vi "route.vi"() -> ()   [LabVIEW 2014]
uses:
  <vilib>/Utility/sysdir.llb/System Directory Type.ctl
  <vilib>/Utility/config.llb/Read Key (Path).vi
  <vilib>/Utility/file.llb/Write To Spreadsheet File (string).vi
  <vilib>/Utility/config.llb/Write Key (Path).vi
  <vilib>/httpClient/LabVIEWHTTPClient.lvlib
  <vilib>/Utility/config.llb/NI_LVConfig.lvlib
panel:
  out "FUEL/연료":i32
  out "time/시간":dbl
  in  "도움말":bool
  in  "피드백":bool
  in  "저장 경로":path
  out "Distance":string="0"
  in  "찾기":bool
  in  "?":bool
  in  "?":bool
  out "x fmc 플랜":string
  out "FMS 플랜":string
  in  "Destination":string
  in  "departure":string
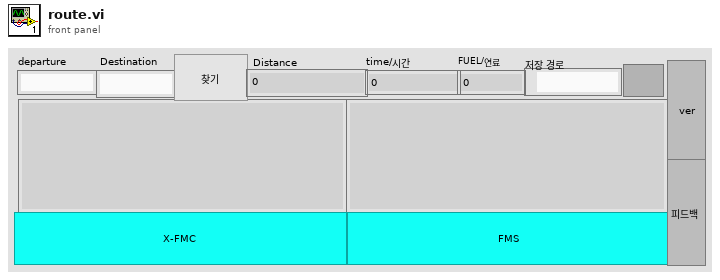
[diagram p1: front panel]
types:
  T1 = enum16{"open", "replace", "create", "open or create", "replace or create", "replace or create with confirmation"}
  T2 = typedef "System Directory Type.ctl" = i32
  T3 = typedef "NI_LVConfig.lvlib/Config Data RefNum.ctl" = refnum<k1>
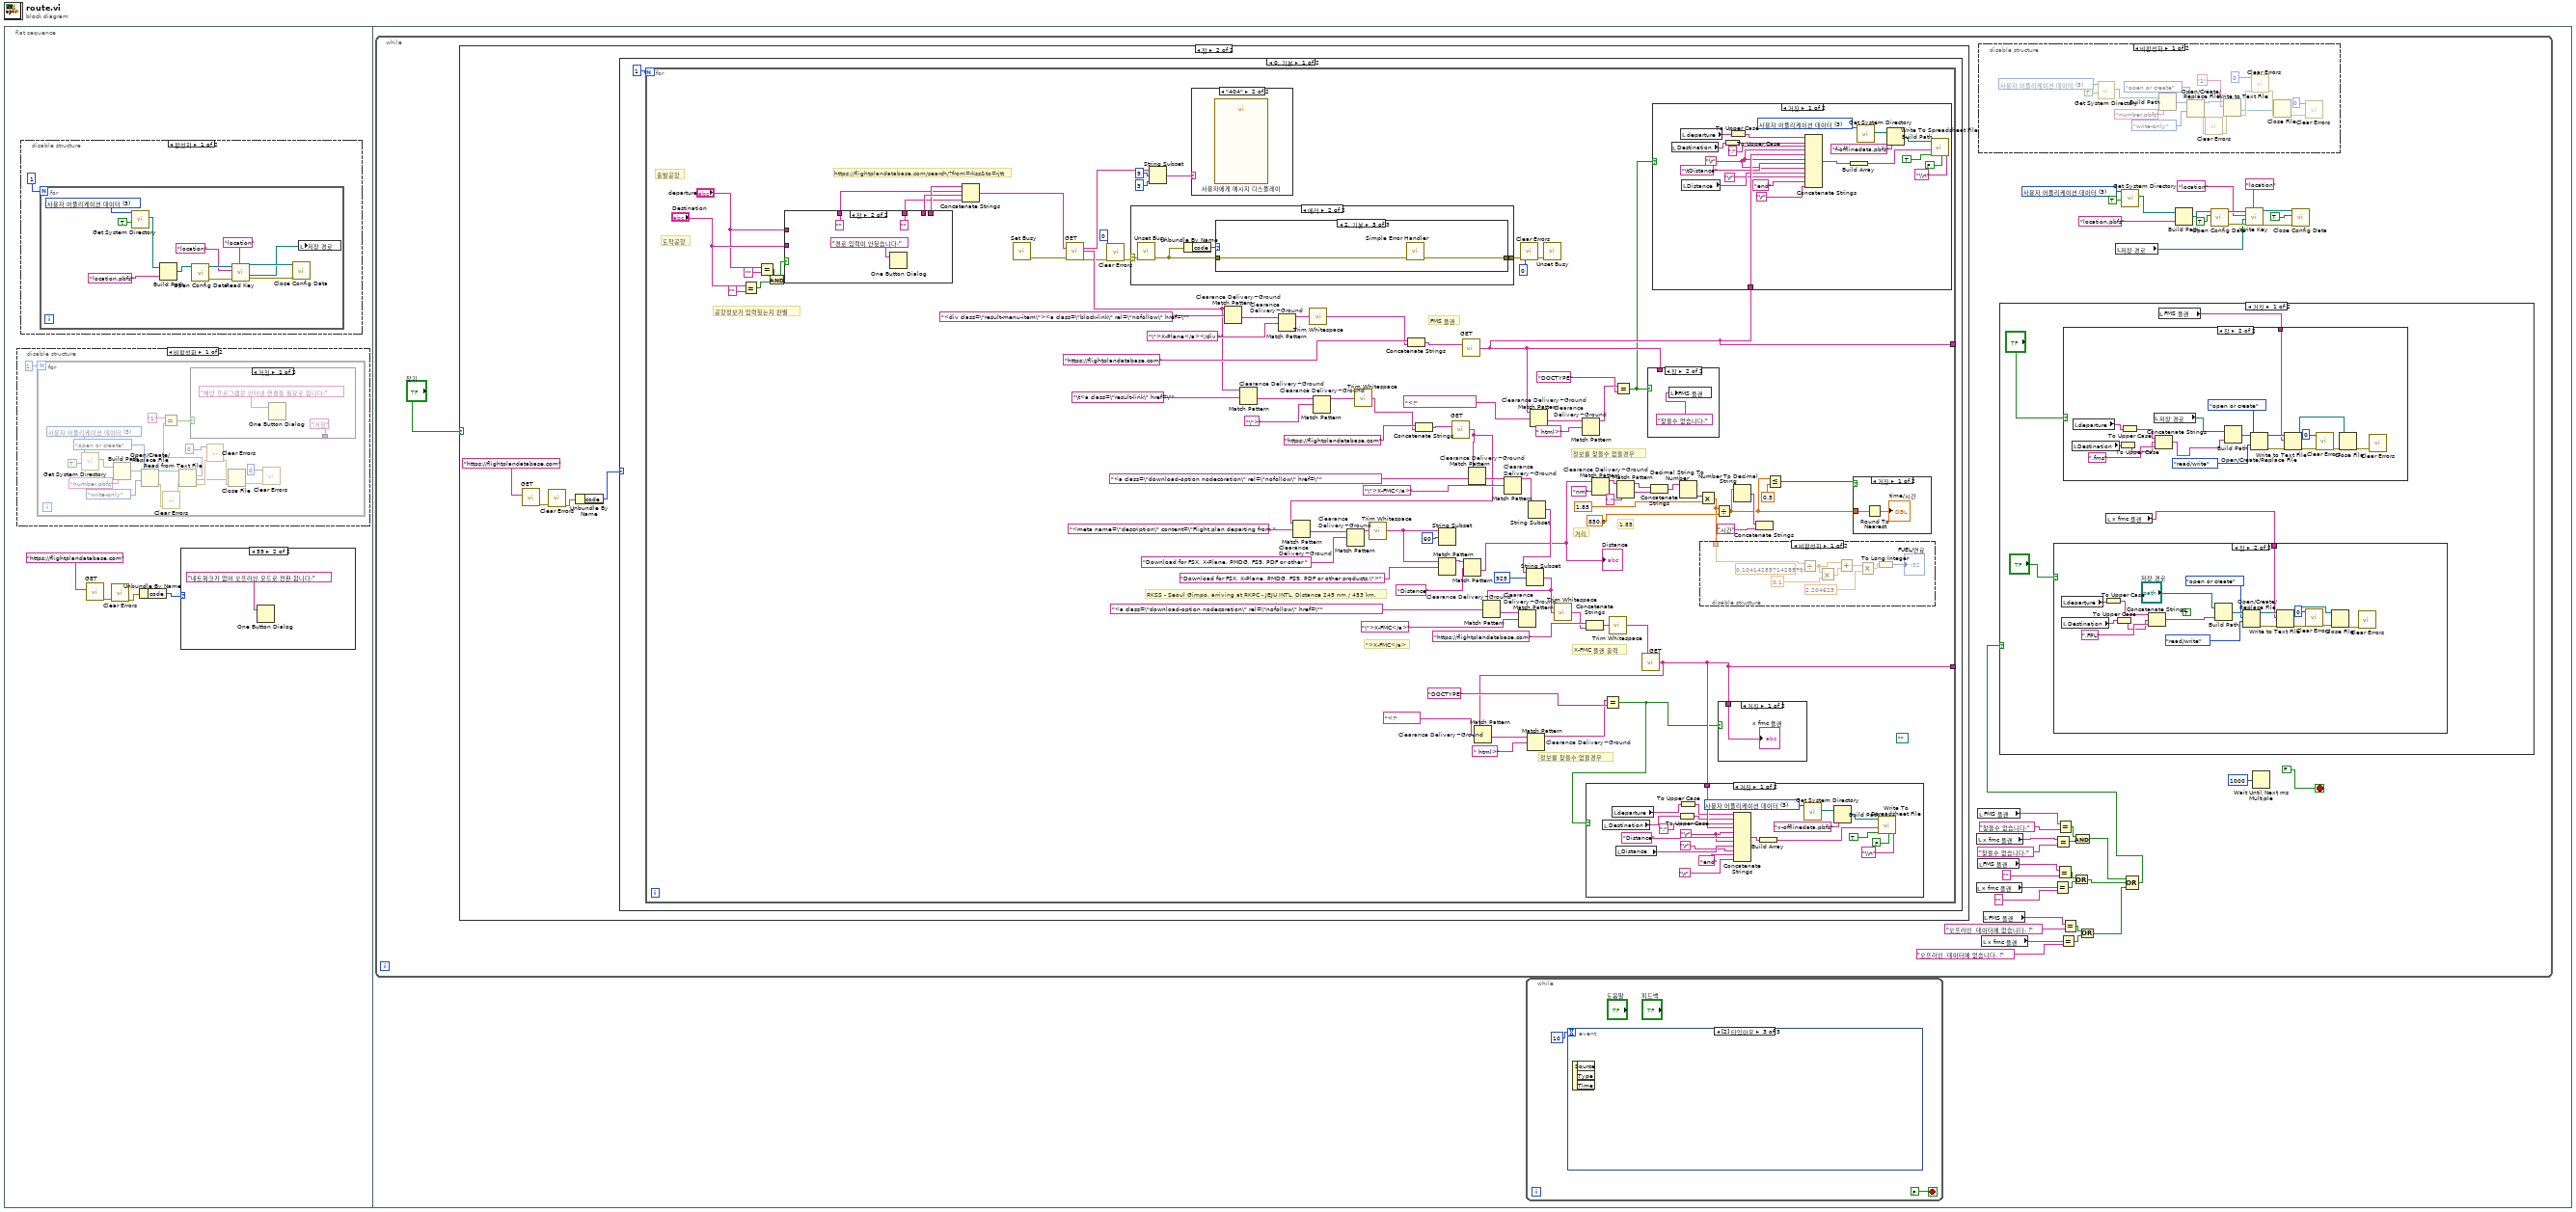
[diagram p0: block diagram]
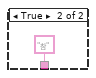
[diagram p3: hidden frame]
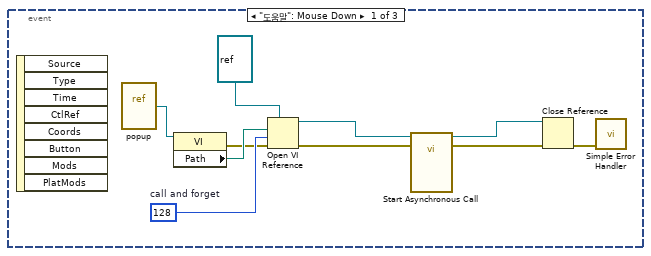
[diagram p6: hidden frame]
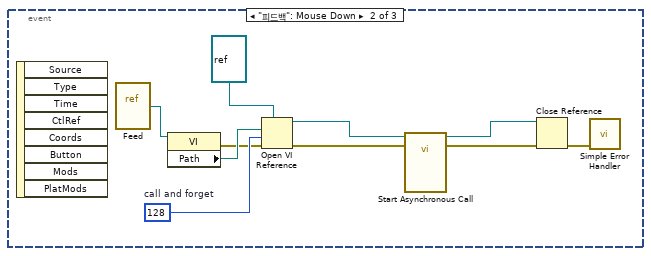
[diagram p7: hidden frame]
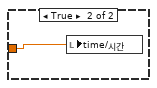
[diagram p12: hidden frame]
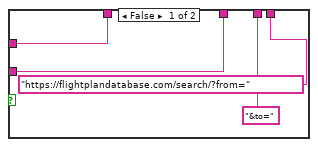
[diagram p13: hidden frame]
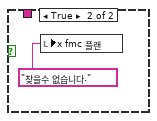
[diagram p14: hidden frame]
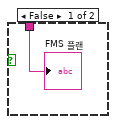
[diagram p15: hidden frame]
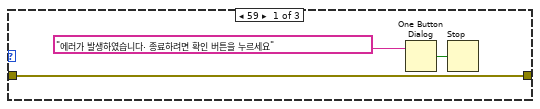
[diagram p18: hidden frame]
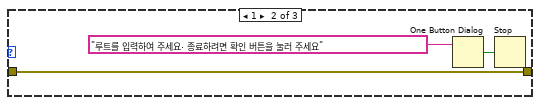
[diagram p19: hidden frame]
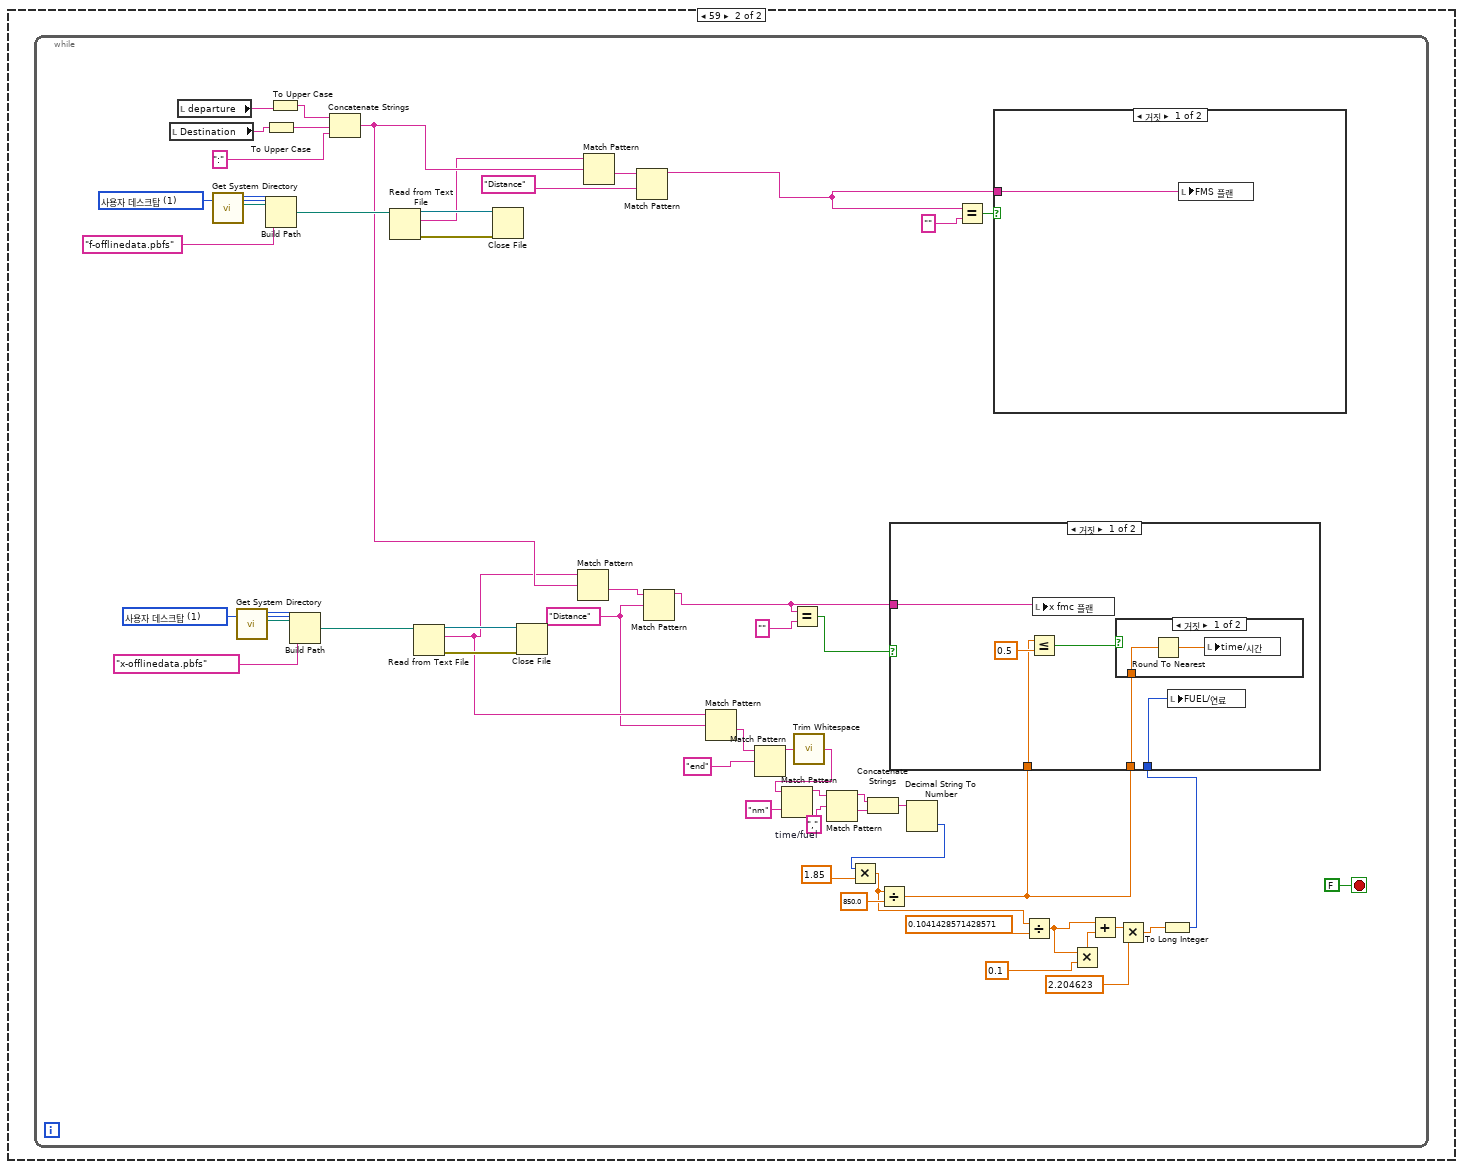
[diagram p20: hidden frame]
diagram:
  n1 = flat-sequence {
    frame #0 {
      n2 = disable-structure shown="비활성화" {
        frame Disabled {
          n3 = for {
            N: 1 -> [_]
            w12 = T2 3 items=["사용자 홈"=0, "사용자 데스크탑"=1, "사용자 문서"=2, "사용자 어플리케이션 데이터"=3, "사용자 환경"=4, "사용자 임시"=5, "퍼블릭 문서"=6, "퍼블릭 어플리케이션 데이터"=7, "퍼블릭 환경"=8, "퍼블릭 캐시"=13, "시스템 코어 라이브러리"=9, "시스템 설치된 라이브러리"=10, "어플리케이션 파일"=11, "부팅 볼륨 루트"=12] ("system directory type")
            n4 = call <vilib>:"Get System Directory.vi"("create directory if not found? (F)"=TRUE, "system directory type"=w12) -> ("system directory"=w13:path)  [unwired: 9 in]
            n5 = Build Path(base path=w13, name or relative path="number.pbfs" ("이름 또는 상대 경로")) -> (appended path=w18:path)
            n6 = Open/Create/Replace File(file path (use dialog)=w18, operation (0:open)=T1."open or create" ("동작(0:open)"), access (0:read/write)=enum16{"read/write", "read-only", "write-only"}."write-only" ("접근(0:읽기/쓰기)")) -> (refnum out=w21:refnum<file>, error out=w10:errorcluster)  [unwired: 3 in, 1 out]
            n7 = call <vilib>:"Clear Errors.vi"("error in (no error)"=w10) -> ("error out"=w9:errorcluster)  [unwired: 5 in, 1 out]
            n8 = Read from Text File(file (use dialog)=w21, error in=w9) -> (refnum out=w22:refnum<file>, text=w7:string, error out=w23:errorcluster)  [unwired: 2 in, 1 out]
            n9 = Equal?(x="1" ("y"), y=w7) -> (x = y?=w17:bool)
            n10 = case shown="거짓" w17 {
              tunnel: ["거짓" "참"] -> _
              frame False {
                n11 = One Button Dialog(message="해당 프로그램은 인터넷 연결을 필요로 합니다." ("메시지")) -> ()  [unwired: 1 in, 1 out]
              }
              frame True {
              }
            }
            n12 = call <vilib>:"Clear Errors.vi"("error in (no error)"=w23, "specific error code to clear (0: all)"=0) -> ("error out"=w24:errorcluster)  [unwired: 4 in, 1 out]
            n13 = Close File(refnum=w22, error in=w24) -> (error out=w15:errorcluster)  [unwired: 1 out]
            n14 = call <vilib>:"Clear Errors.vi"("error in (no error)"=w15, "specific error code to clear (0: all)"=0) -> ()  [unwired: 4 in, 2 out]
          }
        }
        frame Enabled {
        }
      }
      n15 = disable-structure shown="활성화" {
        frame Enabled {
          n16 = for {
            N: 1 -> [_]
            w40 = T2 3 items=["사용자 홈"=0, "사용자 데스크탑"=1, "사용자 문서"=2, "사용자 어플리케이션 데이터"=3, "사용자 환경"=4, "사용자 임시"=5, "퍼블릭 문서"=6, "퍼블릭 어플리케이션 데이터"=7, "퍼블릭 환경"=8, "퍼블릭 캐시"=13, "시스템 코어 라이브러리"=9, "시스템 설치된 라이브러리"=10, "어플리케이션 파일"=11, "부팅 볼륨 루트"=12] ("system directory type")
            n17 = call <vilib>:"Get System Directory.vi"("create directory if not found? (F)"=TRUE, "system directory type"=w40) -> ("system directory"=w38:path)  [unwired: 9 in]
            n18 = Build Path(base path=w38, name or relative path="location.pbfs" ("문자열")) -> (appended path=w37:path)
            n19 = call <vilib>:"Open Config Data.vi"("configuration file path"=w37) -> ("error out"=w34:errorcluster, "refnum"=w33:T3)  [unwired: 8 in, 1 out]
            n20 = call-poly <vilib>:"Read Key.vi"("section"="location", "error in (no error)"=w34, "key"="location", "refnum"=w33) -> ("error out"=w35:errorcluster, "value"=w30:path, "refnum out"=w36:T3)  [unwired: 4 in, 1 out]
            n21 = call <vilib>:"Close Config Data.vi"("error in (no error)"=w35, "refnum"=w36) -> ()  [unwired: 8 in, 2 out]
            n22 = local write "저장 경로"(w30) -> ()
          }
        }
        frame Disabled {
        }
      }
      n23 = call <vilib>:"GET.vi"("url"="https://flightplandatabase.com") -> ("error out"=w4:errorcluster)  [unwired: 11 in, 3 out]
      n24 = call <vilib>:"Clear Errors.vi"("error in (no error)"=w4) -> ("error out"=w2:errorcluster)  [unwired: 5 in, 1 out]
      n25 = Unbundle By Name(w2) -> ("code"=w1:i32)
      n26 = case shown="59" w1 {
        frame 0, Default {
        }
        frame 59 {
          n27 = One Button Dialog(message="네트워크가 없어 오프라인 모드로 전환 합니다." ("메시지")) -> ()  [unwired: 1 in, 1 out]
        }
      }
    }
    frame #1 {
      n28 = while {
        stop <- FALSE stop-if-true
        w84 = T2 3 items=["사용자 홈"=0, "사용자 데스크탑"=1, "사용자 문서"=2, "사용자 어플리케이션 데이터"=3, "사용자 환경"=4, "사용자 임시"=5, "퍼블릭 문서"=6, "퍼블릭 어플리케이션 데이터"=7, "퍼블릭 환경"=8, "퍼블릭 캐시"=13, "시스템 코어 라이브러리"=9, "시스템 설치된 라이브러리"=10, "어플리케이션 파일"=11, "부팅 볼륨 루트"=12] ("system directory type")
        n29 = case shown="참" "찾기" {
          frame False {
          }
          frame True {
            n30 = call <vilib>:"GET.vi"("url"="https://flightplandatabase.com") -> ("error out"=w106:errorcluster)  [unwired: 11 in, 3 out]
            n31 = call <vilib>:"Clear Errors.vi"("error in (no error)"=w106) -> ("error out"=w104:errorcluster)  [unwired: 5 in, 1 out]
            n32 = Unbundle By Name(w104) -> ("code"=w103:i32)
            n33 = case shown="0, 기본" w103 {
              frame 0, Default {
                n34 = for {
                  N: 1 -> [_]
                  tunnel: [w111] -> _
                  tunnel: [w109] -> _
                  (unwired) path ""
                  # "1.85"
                  # "RKSS - Seoul Gimpo, arriving at RKPC - JEJU INTL. Distance 245 nm / 453 km."
                  # "\">X-FMC</a>"
                  # "https://flightplandatabase.com/search/?from=rkss&to=rjtt"
                  # "FMS 플랜"
                  # "거리"
                  # "X-FMC 플랜 출력"
                  # "정보를 찾을수 없을경우"
                  # "정보를 찾을수 없을경우"
                  # "공항정보가 입력됫는지 판별"
                  # "도착공항"
                  # "출발공항"
                  n35 = Equal?(x="Destination", y="") -> (x = y?=w139:bool)
                  n36 = Equal?(x="departure", y="") -> (x = y?=w138:bool)
                  n37 = And(x=w138, y=w139) -> (x .and. y?=w140:bool)
                  n38 = case shown="참" w140 {
                    tunnel: ["&to=" ("문자열") _] -> w129
                    tunnel: ["https://flightplandatabase.com/search/?from=" ("문자열") _] -> w128
                    tunnel: "Destination" -> [w255 _]
                    tunnel: [w255 "" ("Destination")] -> w126
                    tunnel: [w254 "" ("departure")] -> w124
                    tunnel: "departure" -> [w254 _]
                    frame False {
                    }
                    frame True {
                      n39 = One Button Dialog(message="경로 입력이 안됫습니다." ("메시지")) -> ()  [unwired: 1 in, 1 out]
                    }
                  }
                  n40 = Concatenate Strings(w128, w124, w129, w126) -> (w190:string)
                  n41 = call <vilib>:"Set Busy.vi"() -> ("error out"=w195:errorcluster)  [unwired: 10 in, 1 out]
                  n42 = call <vilib>:"GET.vi"("url"=w190, "error in (no error)"=w195) -> ("headers"=w199:string, "body"=w166:string, "error out"=w149:errorcluster)  [unwired: 10 in, 1 out]
                  n43 = call <vilib>:"Clear Errors.vi"("error in (no error)"=w149, "specific error code to clear (0: all)"=0) -> ("error out"=w150:errorcluster)  [unwired: 4 in, 1 out]
                  n44 = case shown="에러" w150 {
                    selector: w150 -> [w265 w268]
                    tunnel: [w265 w266] -> w146
                    frame No Error {
                    }
                    frame Error {
                      n45 = call <vilib>:"Unset Busy.vi"("error in (no error)"=w268) -> ("error out"=w267:errorcluster)  [unwired: 10 in]
                      n46 = Unbundle By Name(w267) -> ("code"=w269:i32)
                      n47 = case shown="2, 기본" w269 {
                        tunnel: w267 -> [w270 w275 w277]
                        tunnel: [w270 w275 w276] -> w266
                        frame 59 {
                          n48 = One Button Dialog(message="에러가 발생하였습니다. 종료하려면 확인 버튼을 누르세요" ("메시지")) -> (true=w271:bool)  [unwired: 1 in]
                          n49 = Stop(stop? (T)=w271) -> ()
                        }
                        frame 1 {
                          n50 = One Button Dialog(message="루트를 입력하여 주세요. 종료하려면 확인 버튼을 눌러 주세요" ("메시지")) -> (true=w273:bool)  [unwired: 1 in]
                          n51 = Stop(stop? (T)=w273) -> ()
                        }
                        frame 2, Default {
                          n52 = call <vilib>:"Simple Error Handler.vi"("error in (no error)"=w277) -> ("error out"=w276:errorcluster)  [unwired: 4 in, 4 out]
                        }
                      }
                    }
                  }
                  n53 = String Subset(string=w199, offset (0)=9 ("오프셋(0)"), length (rest)=3 ("길이(나머지)")) -> (substring=w196:string)
                  n54 = case shown="\"404\"" w196 {
                    frame "거짓", Default {
                    }
                    frame "404" {
                      n55 = call "사용자에게 메시지 디스플레이"() -> ()  [unwired: 10 in, 2 out]
                    }
                  }
                  n56 = Match Pattern "Clearance Delivery~Ground"(string=w166, regular expression="<div class=\"result-menu-item\"><a class=\"block-link\" rel=\"nofollow\" href=\"" ("정규식")) -> (after substring=w193:string)  [unwired: 1 in, 3 out]
                  n57 = Match Pattern "Clearance Delivery~Ground"(string=w166, regular expression="\t<a class=\"result-link\" href=\"" ("정규식")) -> (after substring=w186:string)  [unwired: 1 in, 3 out]
                  n58 = Match Pattern "Clearance Delivery~Ground"(string=w193, regular expression="\">X-Plane</a></div>" ("정규식")) -> (before substring=w191:string)  [unwired: 1 in, 3 out]
                  n59 = call <vilib>:"Trim Whitespace.vi"("string"=w191) -> ("trimmed string"=w187:string)  [unwired: 1 in]
                  n60 = Match Pattern "Clearance Delivery~Ground"(string=w186, regular expression="\">" ("정규식")) -> (before substring=w183:string)  [unwired: 1 in, 3 out]
                  n61 = call <vilib>:"Trim Whitespace.vi"("string"=w183) -> ("trimmed string"=w181:string)  [unwired: 1 in]
                  n62 = Concatenate Strings("https://flightplandatabase.com" ("url"), w187) -> (w188:string)
                  n63 = Concatenate Strings("https://flightplandatabase.com" ("url"), w181) -> (w178:string)
                  n64 = call <vilib>:"GET.vi"("url"=w178) -> ("body"=w164:string)  [unwired: 11 in, 3 out]
                  n65 = Match Pattern "Clearance Delivery~Ground"(string=w164, regular expression="<meta name=\"description\" content=\"Flight plan departing from " ("정규식")) -> (after substring=w167:string)  [unwired: 1 in, 3 out]
                  n66 = Match Pattern "Clearance Delivery~Ground"(string=w167, regular expression="Download for FSX, X-Plane, PMDG, FS9, PDF or other " ("정규식")) -> (before substring=w169:string)  [unwired: 1 in, 3 out]
                  n67 = call <vilib>:"Trim Whitespace.vi"("string"=w169) -> ("trimmed string"=w134:string)  [unwired: 1 in]
                  n68 = String Subset(string=w134, offset (0)=60 ("오프셋(0)")) -> ()  [unwired: 1 in, 1 out]
                  n69 = Match Pattern(string=w134, regular expression="Download for FSX, X-Plane, PMDG, FS9, PDF or other products.\">" ("정규식")) -> (before substring=w132:string)  [unwired: 1 in, 3 out]
                  n70 = call <vilib>:"GET.vi"("url"=w188) -> ("body"=w109:string)  [unwired: 11 in, 3 out]
                  n71 = Match Pattern(string=w132, regular expression="Distance" ("정규식")) -> (after substring=w130:string)  [unwired: 1 in, 3 out]
                  "Distance" <- w130
                  n72 = Match Pattern "Clearance Delivery~Ground"(string=w164, regular expression="<a class=\"download-option nodecoration\" rel=\"nofollow\" href=\"" ("정규식")) -> (after substring=w177:string)  [unwired: 1 in, 3 out]
                  n73 = Match Pattern "Clearance Delivery~Ground"(string=w177, regular expression="\">X-FMC</a>" ("정규식")) -> (before substring=w176:string)  [unwired: 1 in, 3 out]
                  n74 = call <vilib>:"Clear Errors.vi"("error in (no error)"=w146, "specific error code to clear (0: all)"=0) -> ("error out"=w147:errorcluster)  [unwired: 4 in, 1 out]
                  n75 = String Subset(string=w176) -> (substring=w135:string)  [unwired: 2 in]
                  n76 = String Subset(string=w135, offset (0)=925 ("오프셋(0)")) -> (substring=w136:string)  [unwired: 1 in]
                  n77 = Match Pattern "Clearance Delivery~Ground"(string=w136, regular expression="<a class=\"download-option nodecoration\" rel=\"nofollow\" href=\"" ("정규식")) -> (after substring=w173:string)  [unwired: 1 in, 3 out]
                  n78 = Match Pattern "Clearance Delivery~Ground"(string=w173, regular expression="\">X-FMC</a>" ("정규식")) -> ()  [unwired: 1 in, 4 out]
                  n79 = Match Pattern "Clearance Delivery~Ground"(string=w109, regular expression="<!" ("문자열")) -> (after substring=w161:string)  [unwired: 1 in, 3 out]
                  n80 = call <vilib>:"Unset Busy.vi"("error in (no error)"=w147) -> ()  [unwired: 10 in, 1 out]
                  n81 = call <vilib>:"Trim Whitespace.vi"("string"=w136) -> ("trimmed string"=w171:string)  [unwired: 1 in]
                  n82 = Match Pattern "Clearance Delivery~Ground"(string=w161, regular expression=" html>" ("정규식")) -> (before substring=w160:string)  [unwired: 1 in, 3 out]
                  n83 = Concatenate Strings("https://flightplandatabase.com" ("url"), w171) -> (w170:string)
                  n84 = Match Pattern "Clearance Delivery~Ground"(string=w130, regular expression="nm" ("정규식")) -> (before substring=w120:string)  [unwired: 1 in, 3 out]
                  n85 = call <vilib>:"Trim Whitespace.vi"("string"=w170) -> ("trimmed string"=w153:string)  [unwired: 1 in]
                  n86 = Equal?(x=w160, y="DOCTYPE") -> (x = y?=w108:bool)
                  n87 = Match Pattern(string=w120, regular expression="," ("정규식")) -> (before substring=w117:string, after substring=w116:string)  [unwired: 1 in, 2 out]
                  n88 = call <vilib>:"GET.vi"("url"=w153) -> ("body"=w111:string)  [unwired: 11 in, 3 out]
                  n89 = Match Pattern "Clearance Delivery~Ground"(string=w111, regular expression="<!" ("문자열")) -> (after substring=w158:string)  [unwired: 1 in, 3 out]
                  n90 = Match Pattern "Clearance Delivery~Ground"(string=w158, regular expression=" html>" ("정규식")) -> (before substring=w155:string)  [unwired: 1 in, 3 out]
                  n91 = Equal?(x=w155, y="DOCTYPE") -> (x = y?=w110:bool)
                  n92 = case shown="거짓" w110 {
                    tunnel: w111 -> [w240 _]
                    frame False {
                      w234 = "\r"
                      w243 = T2 3 items=["사용자 홈"=0, "사용자 데스크탑"=1, "사용자 문서"=2, "사용자 어플리케이션 데이터"=3, "사용자 환경"=4, "사용자 임시"=5, "퍼블릭 문서"=6, "퍼블릭 어플리케이션 데이터"=7, "퍼블릭 환경"=8, "퍼블릭 캐시"=13, "시스템 코어 라이브러리"=9, "시스템 설치된 라이브러리"=10, "어플리케이션 파일"=11, "부팅 볼륨 루트"=12] ("system directory type")
                      n93 = local read "Destination"() -> (w236:string)
                      n94 = local read "departure"() -> (w239:string)
                      n95 = local read "Distance"() -> (w233:string)
                      n96 = To Upper Case(1:w236) -> (0:w237:string)
                      n97 = To Upper Case(1:w239) -> (0:w238:string)
                      n98 = Concatenate Strings(w238, w237, ":", w240, w234, "Distance" ("문자열"), w234, w233, "\r", "end", "\r") -> (w241:string)
                      n99 = Build Array(w241) -> (w245:string[])
                      n100 = call <vilib>:"Get System Directory.vi"("system directory type"=w243) -> ("system directory"=w247:path)  [unwired: 10 in]
                      n101 = Build Path(base path=w247, name or relative path="x-offlinedata.pbfs" ("이름 또는 상대 경로")) -> (appended path=w246:path)
                      n102 = call-poly <vilib>:"Write To Spreadsheet File.vi"("delimiter (\\t)"="\\n" ("delimiter (\\t)"), "transpose? (no:F)"=FALSE, "append to file? (new file:F)"=TRUE, "1D data"=w245, "file path (dialog if empty)"=w246) -> ()  [unwired: 3 in, 1 out]
                    }
                    frame True {
                    }
                  }
                  n103 = case shown="참" w108 {
                    tunnel: w109 -> [w263 _]
                    frame False {
                      "FMS 플랜" <- w263
                    }
                    frame True {
                      n104 = local write "FMS 플랜"("찾을수 없습니다.") -> ()
                    }
                  }
                  n105 = Concatenate Strings(w117, w116) -> (w119:string)
                  n106 = case shown="거짓" w108 {
                    tunnel: w109 -> [w215 _]
                    frame False {
                      w213 = "\r"
                      w222 = T2 3 items=["사용자 홈"=0, "사용자 데스크탑"=1, "사용자 문서"=2, "사용자 어플리케이션 데이터"=3, "사용자 환경"=4, "사용자 임시"=5, "퍼블릭 문서"=6, "퍼블릭 어플리케이션 데이터"=7, "퍼블릭 환경"=8, "퍼블릭 캐시"=13, "시스템 코어 라이브러리"=9, "시스템 설치된 라이브러리"=10, "어플리케이션 파일"=11, "부팅 볼륨 루트"=12] ("system directory type")
                      n107 = local read "Destination"() -> (w216:string)
                      n108 = local read "departure"() -> (w218:string)
                      n109 = local read "Distance"() -> (w212:string)
                      n110 = To Upper Case(1:w216) -> (0:w217:string)
                      n111 = To Upper Case(1:w218) -> (0:w219:string)
                      n112 = Concatenate Strings(w219, w217, ":", w213, w215, w213, "\tDistance", w213, w212, "\r", "end", "\r") -> (w220:string)
                      n113 = Build Array(w220) -> (w224:string[])
                      n114 = call <vilib>:"Get System Directory.vi"("system directory type"=w222) -> ("system directory"=w226:path)  [unwired: 10 in]
                      n115 = Build Path(base path=w226, name or relative path="f-offlinedata.pbfs" ("이름 또는 상대 경로")) -> (appended path=w225:path)
                      n116 = call-poly <vilib>:"Write To Spreadsheet File.vi"("delimiter (\\t)"="\\n" ("delimiter (\\t)"), "transpose? (no:F)"=FALSE, "append to file? (new file:F)"=TRUE, "1D data"=w224, "file path (dialog if empty)"=w225) -> ()  [unwired: 3 in, 1 out]
                    }
                    frame True {
                    }
                  }
                  n117 = Decimal String To Number(string=w119) -> (number=w121:i32)  [unwired: 2 in, 1 out]
                  n118 = Multiply(x=w121, y=1.85) -> (x*y=w112:dbl)
                  n119 = disable-structure shown="비활성화" {
                    disable-tunnel: w112 -> [w205 _]
                    frame Disabled {
                      n120 = Divide(x=w205, y=0.1041428571428571) -> (x/y=w206:dbl)
                      n121 = Multiply(x=w206, y=0.1) -> (x*y=w204:dbl)
                      n122 = Add(x=w206, y=w204) -> (x+y=w203:dbl)
                      n123 = Multiply(x=w203, y=2.204623) -> (x*y=w200:dbl)
                      n124 = To Long Integer(number=w200) -> (32bit integer=→"FUEL/연료":i32)
                    }
                    frame Enabled {
                    }
                  }
                  n125 = Divide(x=w112, y=850.0) -> (x/y=w113:dbl)
                  n126 = case shown="거짓" w110 {
                    tunnel: w111 -> [w261 _]
                    frame False {
                      "x fmc 플랜" <- w261
                    }
                    frame True {
                      n127 = local write "x fmc 플랜"("찾을수 없습니다.") -> ()
                    }
                  }
                  n128 = Number To Decimal String(number=w113) -> (decimal integer string=w141:string)  [unwired: 1 in]
                  n129 = Concatenate Strings(w141, "시간") -> ()  [unwired: 1 out]
                  n130 = Less Or Equal?(x=w113, y=0.5) -> (x <= y?=w115:bool)
                  n131 = case shown="거짓" w115 {
                    tunnel: w113 -> [w252 w253]
                    frame False {
                      n132 = Round To Nearest(number=w252) -> (nearest integer value=→"time/시간":dbl)
                    }
                    frame True {
                      n133 = local write "time/시간"(w253) -> ()
                    }
                  }
                }
              }
              frame 59 {
                n134 = while {
                  stop <- FALSE stop-if-true
                  w278 = "Distance" ("정규식")
                  w315 = T2 1 items=["사용자 홈"=0, "사용자 데스크탑"=1, "사용자 문서"=2, "사용자 어플리케이션 데이터"=3, "사용자 환경"=4, "사용자 임시"=5, "퍼블릭 문서"=6, "퍼블릭 어플리케이션 데이터"=7, "퍼블릭 환경"=8, "퍼블릭 캐시"=13, "시스템 코어 라이브러리"=9, "시스템 설치된 라이브러리"=10, "어플리케이션 파일"=11, "부팅 볼륨 루트"=12] ("system directory type")
                  w329 = T2 1 items=["사용자 홈"=0, "사용자 데스크탑"=1, "사용자 문서"=2, "사용자 어플리케이션 데이터"=3, "사용자 환경"=4, "사용자 임시"=5, "퍼블릭 문서"=6, "퍼블릭 어플리케이션 데이터"=7, "퍼블릭 환경"=8, "퍼블릭 캐시"=13, "시스템 코어 라이브러리"=9, "시스템 설치된 라이브러리"=10, "어플리케이션 파일"=11, "부팅 볼륨 루트"=12] ("system directory type")
                  n135 = local read "Destination"() -> (w309:string)
                  n136 = local read "departure"() -> (w311:string)
                  n137 = call <vilib>:"Get System Directory.vi"("system directory type"=w315) -> ("system directory"=w314:path)  [unwired: 10 in]
                  n138 = call <vilib>:"Get System Directory.vi"("system directory type"=w329) -> ("system directory"=w330:path)  [unwired: 10 in]
                  n139 = To Upper Case(1:w309) -> (0:w308:string)
                  n140 = Build Path(base path=w314, name or relative path="f-offlinedata.pbfs" ("이름 또는 상대 경로")) -> (appended path=w317:path)
                  n141 = To Upper Case(1:w311) -> (0:w310:string)
                  n142 = Build Path(base path=w330, name or relative path="x-offlinedata.pbfs" ("이름 또는 상대 경로")) -> (appended path=w327:path)
                  n143 = Concatenate Strings(w310, w308, ":") -> (w305:string)
                  n144 = Read from Text File(file (use dialog)=w317) -> (refnum out=w318:refnum<file>, text=w303:string, error out=w319:errorcluster)  [unwired: 3 in, 1 out]
                  n145 = Read from Text File(file (use dialog)=w327) -> (refnum out=w326:refnum<file>, text=w279:string, error out=w325:errorcluster)  [unwired: 3 in, 1 out]
                  n146 = Close File(refnum=w318, error in=w319) -> ()  [unwired: 2 out]
                  n147 = Close File(refnum=w326, error in=w325) -> ()  [unwired: 2 out]
                  n148 = Match Pattern(string=w279, regular expression=w305) -> (after substring=w307:string)  [unwired: 1 in, 3 out]
                  n149 = Match Pattern(string=w303, regular expression=w305) -> (after substring=w312:string)  [unwired: 1 in, 3 out]
                  n150 = Match Pattern(string=w312, regular expression="Distance") -> (before substring=w313:string)  [unwired: 1 in, 3 out]
                  n151 = Match Pattern(string=w307, regular expression=w278) -> (before substring=w306:string)  [unwired: 1 in, 3 out]
                  n152 = Match Pattern(string=w279, regular expression=w278) -> (after substring=w302:string)  [unwired: 1 in, 3 out]
                  n153 = Match Pattern(string=w302, regular expression="end" ("정규식")) -> (before substring=w292:string)  [unwired: 1 in, 3 out]
                  n154 = Equal?(x=w306, y="") -> (x = y?=w324:bool)
                  n155 = call <vilib>:"Trim Whitespace.vi"("string"=w292) -> ("trimmed string"=w298:string)  [unwired: 1 in]
                  n156 = Match Pattern "time/fuel"(string=w298, regular expression="nm" ("정규식")) -> (before substring=w294:string)  [unwired: 1 in, 3 out]
                  n157 = Match Pattern(string=w294, regular expression="," ("정규식")) -> (before substring=w296:string, after substring=w297:string)  [unwired: 1 in, 2 out]
                  n158 = Concatenate Strings(w296, w297) -> (w295:string)
                  n159 = Decimal String To Number(string=w295) -> (number=w283:i32)  [unwired: 2 in, 1 out]
                  n160 = Multiply(x=w283, y=1.85) -> (x*y=w282:dbl)
                  n161 = Divide(x=w282, y=850.0) -> (x/y=w280:dbl)
                  n162 = Equal?(x=w313, y="") -> (x = y?=w321:bool)
                  n163 = case shown="거짓" w321 {
                    tunnel: w313 -> [w332 _]
                    frame False {
                      n164 = local write "FMS 플랜"(w332) -> ()
                    }
                    frame True {
                      n165 = local write "x fmc 플랜"("오프라인  데이터에 없습니다. !" ("메시지")) -> ()
                    }
                  }
                  n166 = Divide(x=w282, y=0.1041428571428571) -> (x/y=w286:dbl)
                  n167 = Multiply(x=w286, y=0.1) -> (x*y=w287:dbl)
                  n168 = Add(x=w286, y=w287) -> (x+y=w288:dbl)
                  n169 = Multiply(x=w288, y=2.204623) -> (x*y=w290:dbl)
                  n170 = To Long Integer(number=w290) -> (32bit integer=w281:i32)
                  n171 = case shown="거짓" w324 {
                    tunnel: w306 -> [w339 _]
                    tunnel: w281 -> [w334 _]
                    tunnel: w280 -> [w335 _]
                    tunnel: w280 -> [w336 _]
                    frame False {
                      n172 = Less Or Equal?(x=w336, y=0.5) -> (x <= y?=w338:bool)
                      n173 = local write "x fmc 플랜"(w339) -> ()
                      n174 = case shown="거짓" w338 {
                        tunnel: w335 -> [w340 w342]
                        frame False {
                          n175 = Round To Nearest(number=w340) -> (nearest integer value=w341:dbl)
                          n176 = local write "time/시간"(w341) -> ()
                        }
                        frame True {
                          n177 = local write "time/시간"(w342) -> ()
                        }
                      }
                      n178 = local write "FUEL/연료"(w334) -> ()
                    }
                    frame True {
                      n179 = local write "x fmc 플랜"("오프라인  데이터에 없습니다. !" ("메시지")) -> ()
                    }
                  }
                }
              }
            }
          }
        }
        n180 = local read "x fmc 플랜"() -> (w91:string)
        n181 = local read "x fmc 플랜"() -> (w99:string)
        n182 = local read "FMS 플랜"() -> (w86:string)
        n183 = local read "FMS 플랜"() -> (w97:string)
        n184 = disable-structure shown="비활성화" {
          frame Disabled {
            w347 = T2 3 items=["사용자 홈"=0, "사용자 데스크탑"=1, "사용자 문서"=2, "사용자 어플리케이션 데이터"=3, "사용자 환경"=4, "사용자 임시"=5, "퍼블릭 문서"=6, "퍼블릭 어플리케이션 데이터"=7, "퍼블릭 환경"=8, "퍼블릭 캐시"=13, "시스템 코어 라이브러리"=9, "시스템 설치된 라이브러리"=10, "어플리케이션 파일"=11, "부팅 볼륨 루트"=12] ("system directory type")
            n185 = call <vilib>:"Get System Directory.vi"("create directory if not found? (F)"=TRUE, "system directory type"=w347) -> ("system directory"=w348:path)  [unwired: 9 in]
            n186 = Build Path(base path=w348, name or relative path="number.pbfs" ("이름 또는 상대 경로")) -> (appended path=w353:path)
            n187 = Open/Create/Replace File(file path (use dialog)=w353, operation (0:open)=T1."open or create" ("동작(0:open)"), access (0:read/write)=enum16{"read/write", "read-only", "write-only"}."write-only" ("접근(0:읽기/쓰기)")) -> (refnum out=w356:refnum<file>, error out=w345:errorcluster)  [unwired: 3 in, 1 out]
            n188 = call <vilib>:"Clear Errors.vi"("error in (no error)"=w345) -> ("error out"=w344:errorcluster)  [unwired: 5 in, 1 out]
            n189 = Write to Text File(file (use dialog)=w356, text="1" ("텍스트"), error in=w344) -> (refnum out=w357:refnum<file>, error out=w358:errorcluster)  [unwired: 1 in, 1 out]
            n190 = call <vilib>:"Clear Errors.vi"("error in (no error)"=w358, "specific error code to clear (0: all)"=0) -> ("error out"=w359:errorcluster)  [unwired: 4 in, 1 out]
            n191 = Close File(refnum=w357, error in=w359) -> (error out=w350:errorcluster)  [unwired: 1 out]
            n192 = call <vilib>:"Clear Errors.vi"("error in (no error)"=w350, "specific error code to clear (0: all)"=0) -> ()  [unwired: 4 in, 2 out]
          }
          frame Enabled {
          }
        }
        n193 = local read "x fmc 플랜"() -> (w68:string)
        n194 = local read "FMS 플랜"() -> (w64:string)
        n195 = Equal?(x=w91, y="") -> (x = y?=w93:bool)
        n196 = Equal?(x=w99, y="찾을수 없습니다.") -> (x = y?=w100:bool)
        n197 = Equal?(x=w86, y="") -> (x = y?=w92:bool)
        n198 = Equal?(x=w97, y="찾을수 없습니다.") -> (x = y?=w101:bool)
        n199 = Equal?(x=w68, y="오프라인  데이터에 없습니다. !") -> (x = y?=w66:bool)
        n200 = Equal?(x=w64, y="오프라인  데이터에 없습니다. !") -> (x = y?=w67:bool)
        n201 = Or(x=w92, y=w93) -> (x .or. y?=w81:bool)
        n202 = And(x=w101, y=w100) -> (x .and. y?=w88:bool)
        n203 = Or(x=w67, y=w66) -> (x .or. y?=w65:bool)
        n204 = local read "저장 경로"() -> (w72:path)
        n205 = call <vilib>:"Get System Directory.vi"("create directory if not found? (F)"=TRUE, "system directory type"=w84) -> ("system directory"=w82:path)  [unwired: 9 in]
        n206 = Compound Arithmetic op=OR(w88, w81, w65) -> (w87:bool)
        n207 = case shown="거짓" w87 {
          frame False {
            n208 = local read "x fmc 플랜"() -> (w361:string)
            n209 = case shown="참" "?" {
              tunnel: w361 -> [_ w384]
              frame False {
              }
              frame True {
                (unwired) TRUE ("create directory if not found? (F)")
                n210 = local read "departure"() -> (w392:string)
                n211 = local read "Destination"() -> (w391:string)
                n212 = To Upper Case(1:w392) -> (0:w383:string)
                n213 = To Upper Case(1:w391) -> (0:w390:string)
                n214 = Concatenate Strings(w383, w390, ".FPL" ("문자열")) -> (w395:string)
                n215 = Build Path(base path="저장 경로", name or relative path=w395) -> (appended path=w398:path)
                n216 = Open/Create/Replace File(file path (use dialog)=w398, operation (0:open)=T1."open or create" ("동작(0:open)"), access (0:read/write)=enum16{"read/write", "read-only", "write-only"}."read/write" ("접근(0:읽기/쓰기)")) -> (refnum out=w400:refnum<file>, error out=w399:errorcluster)  [unwired: 3 in, 1 out]
                n217 = Write to Text File(file (use dialog)=w400, text=w384, error in=w399) -> (refnum out=w387:refnum<file>, error out=w389:errorcluster)  [unwired: 1 in, 1 out]
                n218 = call <vilib>:"Clear Errors.vi"("error in (no error)"=w389, "specific error code to clear (0: all)"=0) -> ("error out"=w388:errorcluster)  [unwired: 4 in, 1 out]
                n219 = Close File(refnum=w387, error in=w388) -> (error out=w385:errorcluster)  [unwired: 1 out]
                n220 = call <vilib>:"Clear Errors.vi"("error in (no error)"=w385) -> ()  [unwired: 5 in, 2 out]
              }
            }
            n221 = local read "FMS 플랜"() -> (w363:string)
            n222 = case shown="참" "?" {
              tunnel: w363 -> [_ w376]
              frame False {
              }
              frame True {
                n223 = local read "Destination"() -> (w373:string)
                n224 = local read "departure"() -> (w371:string)
                n225 = To Upper Case(1:w373) -> (0:w372:string)
                n226 = To Upper Case(1:w371) -> (0:w365:string)
                n227 = local read "저장 경로"() -> (w367:path)
                n228 = Concatenate Strings(w365, w372, ".fms" ("문자열")) -> (w374:string)
                n229 = Build Path(base path=w367, name or relative path=w374) -> (appended path=w379:path)
                n230 = Open/Create/Replace File(file path (use dialog)=w379, operation (0:open)=T1."open or create" ("동작(0:open)"), access (0:read/write)=enum16{"read/write", "read-only", "write-only"}."read/write" ("접근(0:읽기/쓰기)")) -> (refnum out=w382:refnum<file>, error out=w381:errorcluster)  [unwired: 3 in, 1 out]
                n231 = Write to Text File(file (use dialog)=w382, text=w376, error in=w381) -> (refnum out=w380:refnum<file>, error out=w370:errorcluster)  [unwired: 1 in, 1 out]
                n232 = call <vilib>:"Clear Errors.vi"("error in (no error)"=w370, "specific error code to clear (0: all)"=0) -> ("error out"=w369:errorcluster)  [unwired: 4 in, 1 out]
                n233 = Close File(refnum=w380, error in=w369) -> (error out=w366:errorcluster)  [unwired: 1 out]
                n234 = call <vilib>:"Clear Errors.vi"("error in (no error)"=w366) -> ()  [unwired: 5 in, 2 out]
              }
            }
          }
          frame True {
          }
        }
        n235 = Build Path(base path=w82, name or relative path="location.pbfs" ("문자열")) -> (appended path=w80:path)
        n236 = call <vilib>:"Open Config Data.vi"("create file if necessary (T)"=TRUE, "configuration file path"=w80) -> ("error out"=w78:errorcluster, "refnum"=w77:T3)  [unwired: 7 in, 1 out]
        n237 = call-poly <vilib>:"Write Key.vi"("section"="location", "error in (no error)"=w78, "value"=w72, "key"="location", "refnum"=w77) -> ("error out"=w75:errorcluster, "refnum out"=w76:T3)  [unwired: 4 in, 1 out]
        n238 = Wait Until Next ms Multiple(millisecond multiple=u32 1000 ("ms 배수")) -> ()  [unwired: 1 out]
        n239 = call <vilib>:"Close Config Data.vi"("error in (no error)"=w75, "write file if changed (T)"=TRUE, "refnum"=w76) -> ()  [unwired: 7 in, 2 out]
      }
      n240 = while {
        stop <- FALSE stop-if-true
        n241 = event shown="[2] 타임아웃" {
          selector: _ -> [_ _ _]
          dyn-events: _ -> [_ _ _]
          timeout: 10 -> [_ _ _]
          event "도움말": Mouse Down {
            w53 = 128  # call and forget
            n242 = event-data() -> ()  [unwired: 1 in, 8 out]
            n243 = vi-ref "popup.vi"() -> (w46:refnum<vi>)
            n244 = property class="VI"(reference=w46) -> (error out=w47:errorcluster, "Path"=w48:path)  [unwired: 1 in, 1 out]
            n245 = Open VI Reference(type specifier VI Refnum (for type only)=refnum<vi> refnum, vi path=w48, options=w53, error in (no error)=w47) -> (vi reference=w45:refnum<vi>, error out=w51:errorcluster)  [unwired: 2 in]
            n246 = call-by-ref "Start Asynchronous Call"(reference=w45, error in=w51) -> (reference out=w44:refnum<vi>, error out=w50:errorcluster)  [unwired: 12 in]
            n247 = Close Reference(reference=w44, error in (no error)=w50) -> (error out=w49:errorcluster)
            n248 = call <vilib>:"Simple Error Handler.vi"("error in (no error)"=w49) -> ()  [unwired: 4 in, 5 out]
          }
          event "피드백": Mouse Down {
            w63 = 128  # call and forget
            n249 = event-data() -> ()  [unwired: 1 in, 8 out]
            n250 = vi-ref "Feed.vi"() -> (w56:refnum<vi>)
            n251 = property class="VI"(reference=w56) -> (error out=w57:errorcluster, "Path"=w58:path)  [unwired: 1 in, 1 out]
            n252 = Open VI Reference(type specifier VI Refnum (for type only)=refnum<vi> refnum, vi path=w58, options=w63, error in (no error)=w57) -> (vi reference=w55:refnum<vi>, error out=w61:errorcluster)  [unwired: 2 in]
            n253 = call-by-ref "Start Asynchronous Call"(reference=w55, error in=w61) -> (reference out=w54:refnum<vi>, error out=w60:errorcluster)  [unwired: 12 in]
            n254 = Close Reference(reference=w54, error in (no error)=w60) -> (error out=w59:errorcluster)
            n255 = call <vilib>:"Simple Error Handler.vi"("error in (no error)"=w59) -> ()  [unwired: 4 in, 5 out]
          }
          event Timeout {
            n256 = event-data() -> ()  [unwired: 1 in, 3 out]
          }
        }
      }
    }
  }
